vi "61_Vision_RC Servo.vi"() -> ()   [LabVIEW 2018]
uses:
  <userlib>/KNR OS 4.0 LabVIEW Toolkit/Type Definition/Resource.ctl
  <userlib>/KNR OS 4.0 LabVIEW Toolkit/Type Definition/RC Servo Port.ctl
panel:
  in  "Sensitivity":dbl(slide)=0.5 scale=0.0..2.0
  out "RC Pulse Width (uS)":u16[](array[numeric])
  out "Image Out":T1(plugin-control)
  in  "stop":bool
  # "靈敏度"
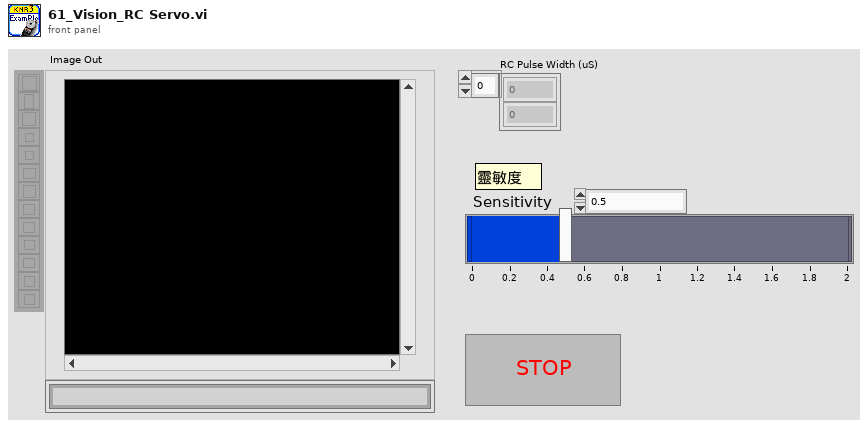
[diagram p1: front panel]
types:
  T1 = typedef "IMAQ Image.ctl" = refnum<image>
  T2 = typedef "RC Servo Port.ctl" = u16
  T3 = typedef "Resource.ctl" = enum16{"KNRm_DDRC", "KNRm_DDDD", "KNRm_DDDR", "KNRm_DDDC", "KNR", "KNRm_neww"}
  T4 = typedef "KNR3 Reference.ctl" = cluster{"FPGA Session":refnum<class "FPGA Interface Base.lvclass">, "Resource":T3}
  T5 = cluster{"Left":dbl, "Top":dbl, "Right":dbl, "Bottom":dbl}
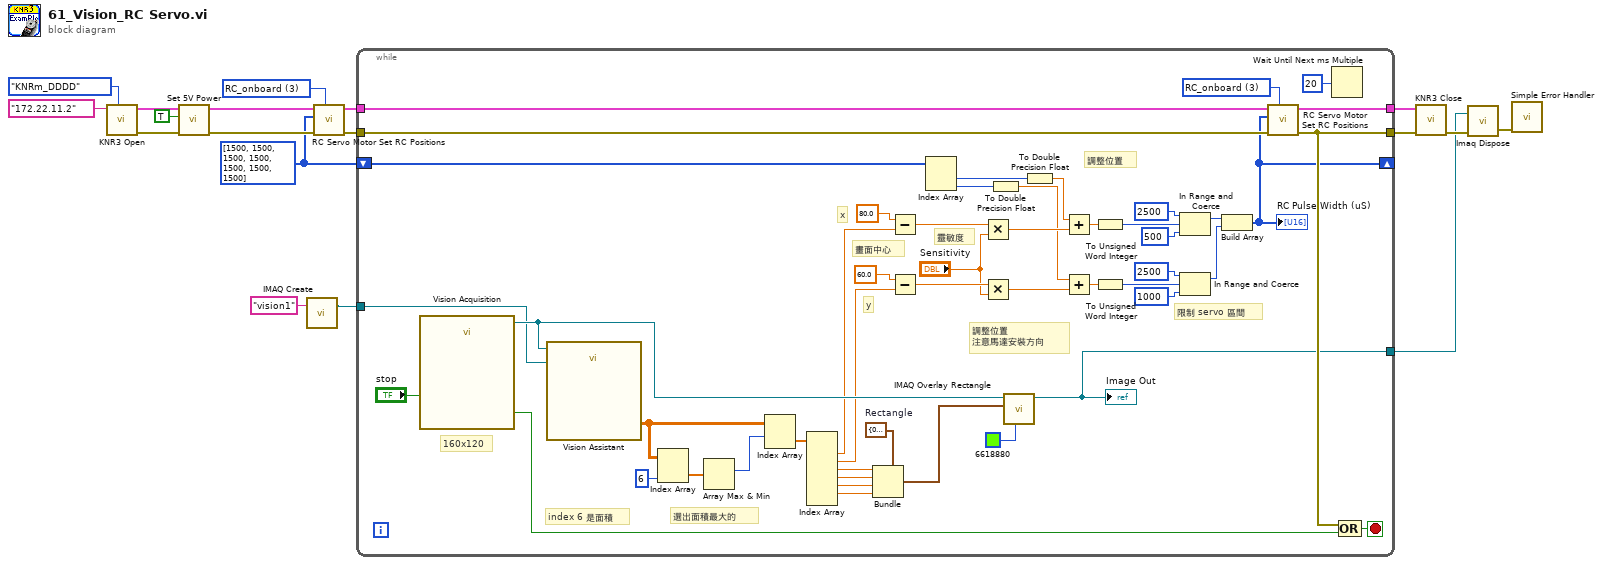
[diagram p0: block diagram]
diagram:
  w4 = u16[] [1500, 1500, 1500, 1500, 1500, 1500, 1500] ("RC Pulse Width (1500 uS)")
  w7 = T2 3 items=["RC_onboard"=3, "RC_box"=9] ("Port (RC_onboard)")
  n1 = call <userlib>:"KNR3 Open.vi"("Resource"=Resource."KNRm_DDDD", "IP"="172.22.11.2") -> ("error out"=w15:errorcluster, "KNR out"=w17:T4)  [unwired: 8 in]
  n2 = call <userlib>:"Set 5V Power.vi"("error in (no error)"=w15, "5V Power(T)"=TRUE ("5V Power"), "KNR in"=w17) -> ("error out"=w14:errorcluster, "KNR out"=w16:T4)  [unwired: 7 in]
  n3 = call "IMAQ Create"("Image Name"="vision1") -> ("New Image"=w5:T1)  [unwired: 4 in, 1 out]
  n4 = call <userlib>:"RC Servo Motor Set RC Positions.vi"("Port (RC_onboard)"=w7, "RC Pulse Width (1500 uS)"=w4, "KNR in"=w16) -> ("KNR out"=w8:T4)  [unwired: 7 in, 1 out]
  n5 = while {
    tunnel: w8 -> [w66]
    tunnel: [w65] -> w10
    tunnel: w14 -> [w64]
    tunnel: [w62] -> w9
    tunnel: w5 -> [w46]
    shift-right: [w30] -> _
    shift-left: w4 -> [w33]
    tunnel: [w18] -> w1
    stop <- w63 stop-if-true
    w58 = T5 {"Left"=0.0, "Top"=0.0, "Right"=0.0, "Bottom"=0.0}  # Rectangle
    w60 = T2 3 items=["RC_onboard"=3, "RC_box"=9] ("RC Motor")
    # "調整位置\n注意馬達安裝方向"
    # "index 6 是面積"
    # "限制 servo 區間"
    # "靈敏度"
    # "畫面中心"
    # "調整位置"
    # "y"
    # "x"
    # "160x120"
    # "選出面積最大的"
    n6 = call "Vision Acquisition"("Stop (F)"="stop") -> ("Image Out"=w51:T1, "Stopped"=w44:bool)  [unwired: 24 in, 1 out]
    n7 = call "Vision Assistant"("Image In"=w51, "Image Dst"=w46) -> ("Particle Measurements (Pixels) (Particle Analysis 1)"=w50:dbl[][])  [unwired: 22 in, 3 out]
    n8 = Index Array "Index Array"(array=w50, index (col)=6 ("disabled index (col)")) -> (element=w49:dbl[])  [unwired: 1 in]
    n9 = Array Max & Min(array=w49) -> (max index (indices)=w48:i32)  [unwired: 3 out]
    n10 = Index Array "Index Array"(array=w50, index (row)=w48) -> (element=w59:dbl[])  [unwired: 1 in]
    n11 = Index Array "Index Array"(array=w59) -> (element #1=w25:dbl, element #2=w24:dbl, element #3=w57:dbl, element #4=w56:dbl, element #5=w55:dbl, element #6=w54:dbl)  [unwired: 7 in, 1 out]
    n12 = Bundle "Bundle"(cluster=w58, "Left"=w57, "Top"=w56, "Right"=w55, "Bottom"=w54) -> (w53:T5)
    n13 = Subtract(x=80.0 ("y"), y=w25) -> (x-y=w40:dbl)
    n14 = Subtract(x=60.0 ("y"), y=w24) -> (x-y=w41:dbl)
    n15 = Index Array "Index Array"(array=w33) -> (element #1=w32:u16, element #2=w31:u16)  [unwired: 2 in]
    n16 = Multiply(x=w40, y="Sensitivity") -> (x*y=w29:dbl)
    n17 = Multiply(x=w41, y="Sensitivity") -> (x*y=w28:dbl)
    n18 = To Double Precision Float(number=w31) -> (double precision float=w20:dbl)
    n19 = call "IMAQ Overlay Rectangle"("Color"=u32 6618880, "Rectangle"=w53, "Image"=w51) -> ("Image Out"=w18:T1)  [unwired: 7 in, 1 out]
    "Image Out" <- w18
    n20 = To Double Precision Float(number=w32) -> (double precision float=w21:dbl)
    n21 = Add(x=w21, y=w29) -> (x+y=w42:dbl)
    n22 = Add(x=w20, y=w28) -> (x+y=w43:dbl)
    n23 = To Unsigned Word Integer(number=w42) -> (unsigned 16bit integer=w23:u16)
    n24 = To Unsigned Word Integer(number=w43) -> (unsigned 16bit integer=w22:u16)
    n25 = In Range and Coerce(upper limit=u16 2500, x=w23, lower limit=u16 500) -> (coerced(x)=w38:u16)  [unwired: 1 out]
    n26 = In Range and Coerce(upper limit=u16 2500, x=w22, lower limit=u16 1000) -> (coerced(x)=w39:u16)  [unwired: 1 out]
    n27 = Build Array(w38, w39) -> (w30:u16[])
    "RC Pulse Width (uS)" <- w30
    n28 = call <userlib>:"RC Servo Motor Set RC Positions.vi"("Port (RC_onboard)"=w60, "error in (no error)"=w64, "RC Pulse Width (1500 uS)"=w30, "KNR in"=w66) -> ("error out"=w62:errorcluster, "KNR out"=w65:T4)  [unwired: 6 in]
    n29 = Wait Until Next ms Multiple(millisecond multiple=u32 20) -> ()  [unwired: 1 out]
    n30 = Compound Arithmetic op=OR(w62, w44) -> (w63:bool)
  }
  n31 = call <userlib>:"KNR3 Close.vi"("error in (no error)"=w9, "KNR in"=w10) -> ("error out"=w3:errorcluster)  [unwired: 9 in]
  n32 = call "Imaq Dispose"("Image"=w1, "error in (no error)"=w3) -> ("error out"=w2:errorcluster)  [unwired: 4 in]
  n33 = call <vilib>:"Simple Error Handler.vi"("error in (no error)"=w2) -> ()  [unwired: 4 in, 5 out]
